vi "Variant to String.vi"(8 "error in (no error)":errorcluster, 10 "Variant":variant, 11 "Timestamp Value in":refnum<class "Timestamp Value.lvclass">) -> (0 "error out":errorcluster, 2 "String":string, 3 "Timestamp Value out":refnum<class "Timestamp Value.lvclass">)   [LabVIEW 2020, in "Composed Columns.lvlib" / "Timestamp Value.lvclass"]
uses:
  Timestamp Value.lvclass
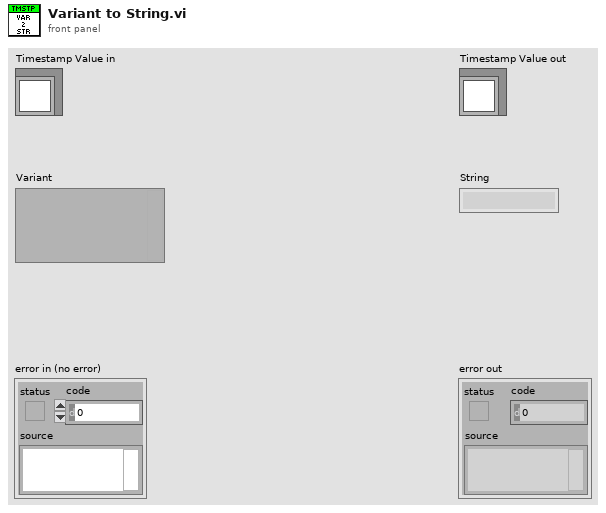
[diagram p1: front panel]
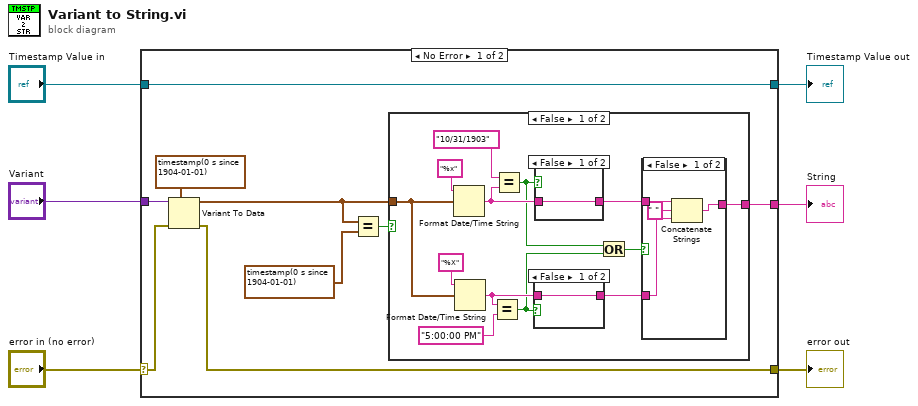
[diagram p0: block diagram]
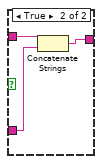
[diagram p2: hidden frame]
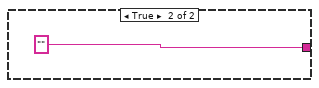
[diagram p5: hidden frame]
diagram:
  n1 = case shown="No Error" "error in (no error)" {
    selector: "error in (no error)" -> [w9 w40]
    tunnel: [w8 w40] -> w5
    tunnel: "Timestamp Value in" -> [w10 w39]
    tunnel: [w10 w39] -> w3
    tunnel: "Variant" -> [w13 _]
    tunnel: [w7 _] -> w1
    frame No Error {
      n2 = Variant To Data(error in=w9, type=timestamp(0 s since 1904-01-01) ("Time Stamp"), Variant=w13) -> (data=w11:timestamp, error out=w8:errorcluster)
      n3 = Equal?(x=w11, y=timestamp(0 s since 1904-01-01) ("Time Stamp")) -> (x = y?=w15:bool)
      n4 = case shown="False" w15 {
        tunnel: [w16 "" ("date/time string")] -> w7
        tunnel: w11 -> [w26 _]
        frame False {
          n5 = Format Date/Time String(time format string (%c)="%x" ("format string"), seconds (now)=w26) -> (date/time string=w24:string)  [unwired: 1 in]
          n6 = Format Date/Time String(time format string (%c)="%X" ("format string"), seconds (now)=w26) -> (date/time string=w25:string)  [unwired: 1 in]
          n7 = Equal?(x=w25, y="5:00:00 PM") -> (x = y?=w19:bool)
          n8 = Equal?(x="10/31/1903", y=w24) -> (x = y?=w20:bool)
          n9 = case shown="False" w19 {
            tunnel: w25 -> [w37 _]
            tunnel: [w37 _] -> w17
            frame False {
            }
            frame True {
            }
          }
          n10 = case shown="False" w20 {
            tunnel: w24 -> [w36 _]
            tunnel: [w36 _] -> w18
            frame False {
            }
            frame True {
            }
          }
          n11 = Or(x=w20, y=w19) -> (x .or. y?=w21:bool)
          n12 = case shown="False" w21 {
            tunnel: w18 -> [w32 w34]
            tunnel: w17 -> [w31 w33]
            tunnel: [w29 w35] -> w16
            frame False {
              n13 = Concatenate Strings(w32, " " ("string"), w31) -> (w29:string)
            }
            frame True {
              n14 = Concatenate Strings(w34, w33) -> (w35:string)
            }
          }
        }
        frame True {
        }
      }
    }
    frame Error {
    }
  }
  "error out" <- w5
  "Timestamp Value out" <- w3
  "String" <- w1
